vi "ScriptEraseFPBP.vi"(8 "error in (no error)":errorcluster, 10 "application reference (local)":refnum<vi>, 11 "VI path":path) -> (0 "error out":errorcluster, 3 "VI out":refnum<vi>)   [LabVIEW 2014]
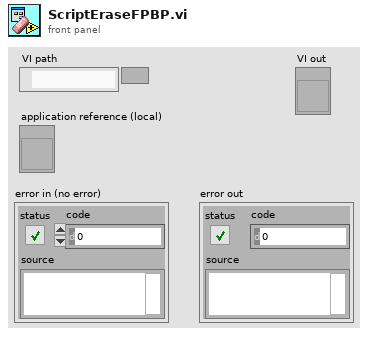
[diagram p1: front panel]
types:
  T1 = enum32{"Invalid", "Standard", "Closed", "Hidden", "Minimized", "Maximized"}
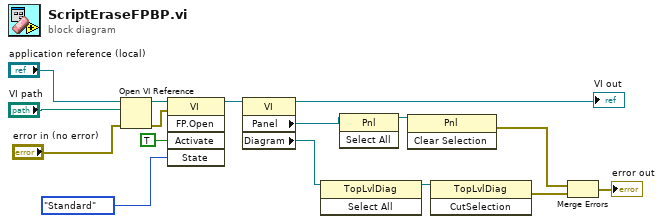
[diagram p0: block diagram]
diagram:
  n1 = Open VI Reference(application reference (local)="application reference (local)", vi path="VI path", error in (no error)="error in (no error)") -> (vi reference=w8:refnum<vi>, error out=w7:errorcluster)  [unwired: 3 in]
  n2 = invoke class="VI" method="FP.Open"(reference=w8, error in=w7, "Activate"=TRUE ("Activate?"), "State"=T1."Standard") -> (reference out=w3:refnum<vi>)  [unwired: 1 in, 4 out]
  n3 = property class="VI"(reference=w3) -> (reference out=→"VI out":refnum<vi>, "Panel"=w15:refnum<vi>, "Diagram"=w16:refnum<vi>)  [unwired: 1 in, 1 out]
  n4 = invoke class="TopLvlDiag" method="Select All"(reference=w16) -> (reference out=w11:refnum<vi>)  [unwired: 2 in, 2 out]
  n5 = invoke class="Pnl" method="Select All"(reference=w15) -> (reference out=w10:refnum<vi>)  [unwired: 2 in, 2 out]
  n6 = invoke class="Pnl" method="Clear Selection"(reference=w10) -> (error out=w14:errorcluster)  [unwired: 2 in, 2 out]
  n7 = invoke class="TopLvlDiag" method="CutSelection"(reference=w11) -> (error out=w12:errorcluster)  [unwired: 2 in, 2 out]
  n8 = Merge Errors(w14, w12) -> (→"error out":errorcluster)
